vi "Format Columns for String.vi"(11 "Column List":string[](array[string])) -> (3 "Column String":string)   [LabVIEW 2017, in "VIs to Interface LabVIEW and MySQL dotNET Connector.lvlib"]
doc: "Convert a list of columns into the correctly formatted string for use in an SQL command"
uses:
  VIs to Interface LabVIEW and MySQL dotNET Connector.lvlib
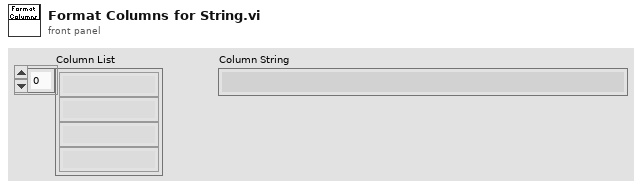
[diagram p1: front panel]
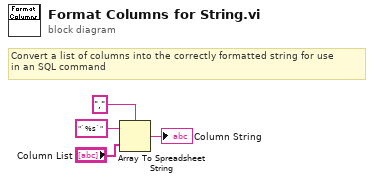
[diagram p0: block diagram]
diagram:
  # "Convert a list of columns into the correctly formatted string for use\nin an SQL command"
  n1 = Array To Spreadsheet String(delimiter (Tab)=",", array="Column List", 3:"`%s`" ("format string")) -> (spreadsheet string=→"Column String":string)
